vi "TCS_spam.vi"() -> ()   [LabVIEW 2011]
uses:
  <vilib>/Instr/_visa.llb/VISA Configure Serial Port (Instr).vi
panel:
  out "moy_aff":dbl format="%.1f"
  out "inst_aff":dbl format="%.3f"
  out "Error":errorcluster
  out "Q String":string
  out "Moyennée":dbl(knob) scale=0.0..5.0
  out "Instantanée":dbl(knob) scale=0.0..5.0
  in  "start":bool
  in  "VISA resource name":refnum<visa-resource-name>
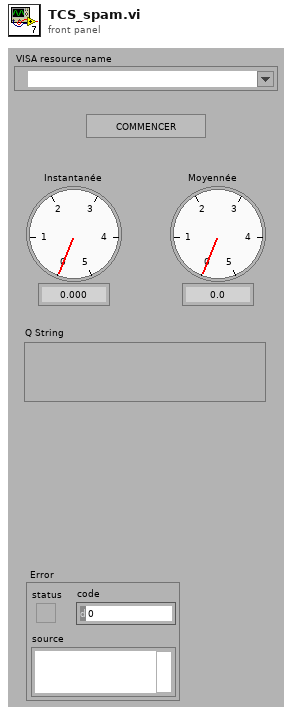
[diagram p1: front panel]
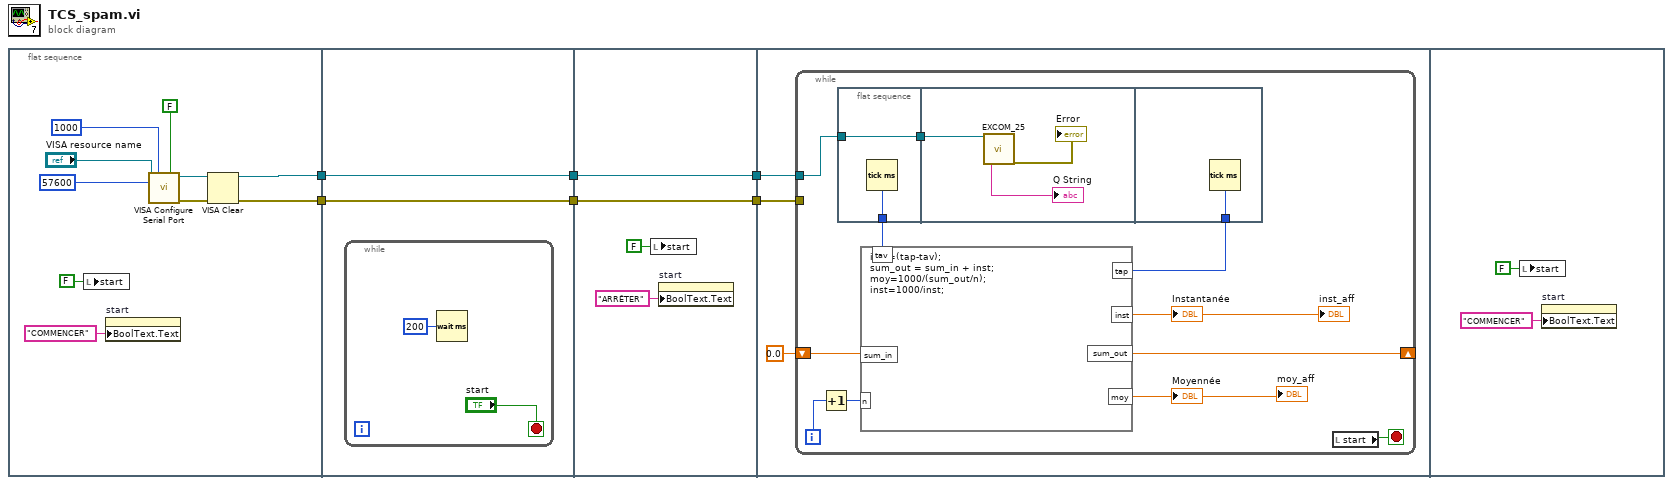
[diagram p0: block diagram]
diagram:
  n1 = flat-sequence {
    tunnel: [w9] -> w5
    tunnel: [w8] -> w3
    tunnel: [w18] -> w6
    tunnel: w5 -> [w18]
    tunnel: [w17] -> w4
    tunnel: w3 -> [w17]
    tunnel: w6 -> [w24]
    tunnel: w4 -> [w23]
    tunnel: [w24] -> w2
    tunnel: [w23] -> w1
    tunnel: w2 -> [w26]
    tunnel: w1 -> [w27]
    frame #0 {
      n2 = local write "start"(FALSE ("start")) -> ()
      n3 = property on="start" class="Bool (strict)"("BoolText.Text"="COMMENCER" ("Boolean Text.Text")) -> ()  [unwired: 2 in, 2 out]
      n4 = call-poly "VISA Configure Serial Port"("VISA resource name"="VISA resource name", "timeout (10sec)"=u32 1000, "Enable Termination\nChar (T)"=FALSE ("Enable Termination\nChar (T)"), "baud rate (9600)"=u32 57600) -> ("VISA resource name out"=w11:refnum<visa-resource-name>, "error out"=w10:errorcluster)  [unwired: 10 in]
      n5 = VISA Clear(VISA resource name=w11, error in (no error)=w10) -> (VISA resource name out=w9:refnum<visa-resource-name>, error out=w8:errorcluster)
    }
    frame #1 {
      n6 = while {
        stop <- "start" stop-if-true
        n7 = Wait (ms)(milliseconds to wait=u32 200) -> ()  [unwired: 1 out]
      }
    }
    frame #2 {
      n8 = local write "start"(FALSE ("start")) -> ()
      n9 = property on="start" class="Bool (strict)"("BoolText.Text"="ARRÊTER" ("Boolean Text.Text")) -> ()  [unwired: 2 in, 2 out]
    }
    frame #3 {
      n10 = while {
        tunnel: w27 -> [_]
        tunnel: w26 -> [w37]
        shift-right: [w30] -> _
        shift-left: 0.0 ("moy") -> [w32]
        i -> [w33]
        stop <- w38 stop-if-true
        n11 = Increment(x=w33) -> (x+1=w31:i32)
        n12 = flat-sequence {
          tunnel: w37 -> [w40]
          tunnel: [w40] -> w36
          tunnel: [w39] -> w35
          tunnel: w36 -> [w42]
          tunnel: [w44] -> w34
          frame #0 {
            n13 = Tick Count (ms)() -> (millisecond timer value=w39:u32)
          }
          frame #1 {
            n14 = call "EXCOM_25.vi"("VISA resource name"=w42) -> ("Q String"=→"Q String":string, "Error OUT"=→"Error":errorcluster)  [unwired: 4 in, 13 out]
          }
          frame #2 {
            n15 = Tick Count (ms)() -> (millisecond timer value=w44:u32)
          }
        }
        n16 = formula code="inst=(tap-tav);\nsum_out = sum_in + inst;\nmoy=1000/(sum_out/n);\ninst=1000/inst;"("tap"=w34, "tav"=w35, "sum_in"=w32, "n"=w31) -> ("inst"=→"Instantanée" →"inst_aff":dbl, "sum_out"=w30:dbl, "moy"=→"Moyennée" →"moy_aff":dbl)
        n17 = local read "start"() -> (w38:bool)
      }
    }
    frame #4 {
      n18 = local write "start"(FALSE ("start")) -> ()
      n19 = property on="start" class="Bool (strict)"("BoolText.Text"="COMMENCER" ("Boolean Text.Text")) -> ()  [unwired: 2 in, 2 out]
    }
  }
